vi "Runmin1.vi"(9 "循环次数 i":i32, 10 "Queue1":T2, 11 "prodatascan":T1) -> (1 "runMin":dbl, 2 "AD":dbl)   [LabVIEW 2018]
uses:
  Initialize/CreateQueue/AllDataQueue.ctl
  Initialize/CreateQueue/SocketQueue.ctl
  Initialize/CreateQueue/LogDataQueue.ctl
  Initialize/CreateQueue/ProDataQueue.ctl
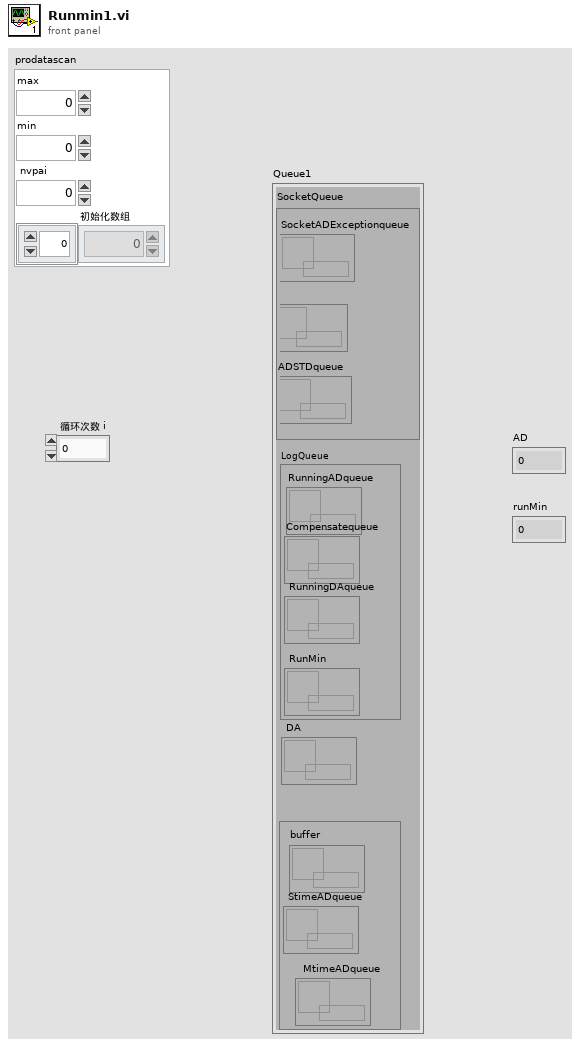
[diagram p1: front panel]
types:
  T1 = cluster{"max":dbl, "min":dbl, " nvpai":dbl, "初始化数组":dbl[]}
  T2 = typedef "AllDataQueue.ctl" = cluster{"SocketQueue":T3, "LogQueue":T4, " DA":refnum<queue>, "ProQueue":T5}
  T3 = typedef "SocketQueue.ctl" = cluster{"ADSTDqueue ":refnum<queue>, "SocketADExceptionqueue":refnum<queue>, "  SocketAD":refnum<queue>}
  T4 = typedef "LogDataQueue.ctl" = cluster{"RunningADqueue":refnum<queue>, "Compensatequeue":refnum<queue>, " RunningDAqueue":refnum<queue>, " RunMin":refnum<queue>}
  T5 = typedef "ProDataQueue.ctl" = cluster{"buffer ":refnum<queue>, " StimeADqueue":refnum<queue>, "  MtimeADqueue":refnum<queue>}
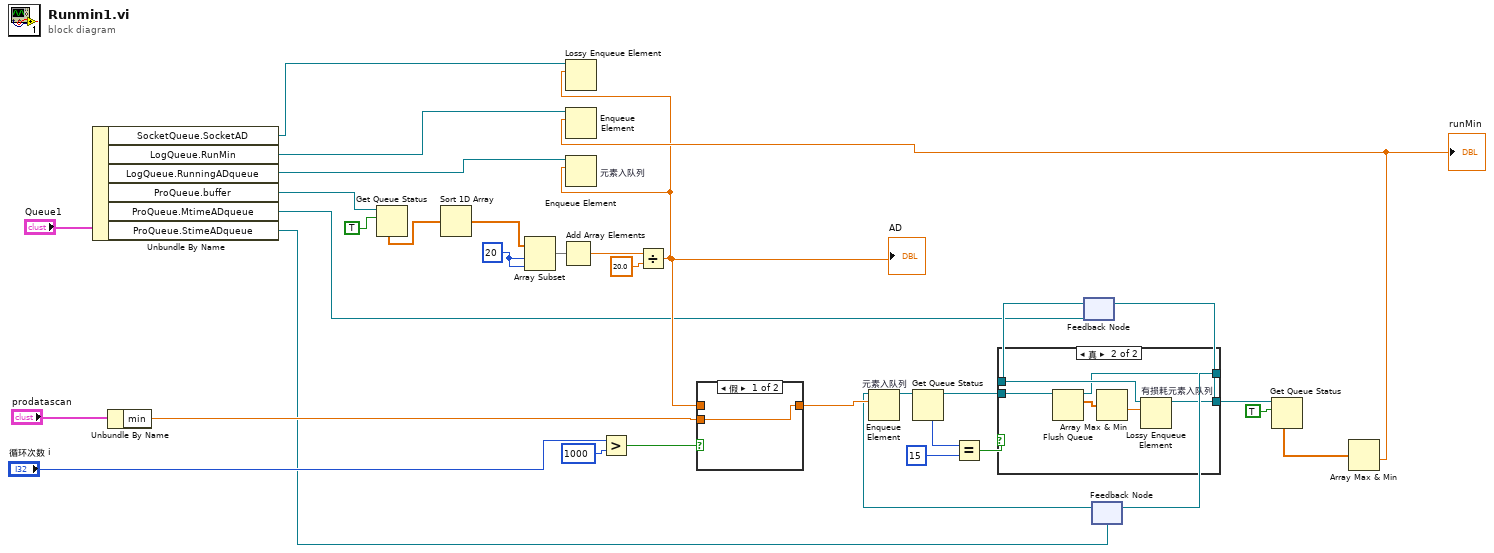
[diagram p0: block diagram]
diagram:
  w3 = 20 ("索引")
  n1 = Unbundle By Name("Queue1") -> ("SocketQueue.SocketAD"=w9:refnum<queue>, "LogQueue.RunMin"=w14:refnum<queue>, "LogQueue.RunningADqueue"=w13:refnum<queue>, "ProQueue.buffer"=w15:refnum<queue>, "ProQueue.MtimeADqueue"=w2:refnum<queue>, "ProQueue.StimeADqueue"=w1:refnum<queue>)
  n2 = Unbundle By Name("prodatascan") -> ("min"=w12:dbl)
  n3 = Get Queue Status(queue=w15, return elements? (F)=TRUE ("返回元素？(F)")) -> (elements=w4:dbl[])  [unwired: 1 in, 7 out]
  n4 = Sort 1D Array(array=w4) -> (sorted array=w10:dbl[])
  n5 = Array Subset(array=w10, index=w3, length=w3) -> (w30:dbl[])
  n6 = Add Array Elements(numeric array=w30) -> (sum=w31:dbl)
  n7 = Greater?(x="循环次数 i", y=1000) -> (0:w27:bool)
  n8 = Divide(x=w31, y=20.0) -> (x/y=w8:dbl)
  "AD" <- w8
  n9 = Lossy Enqueue Element(queue=w9, element=w8) -> ()  [unwired: 1 in, 4 out]
  n10 = Enqueue Element "元素入队列"(queue=w13, element=w8) -> ()  [unwired: 2 in, 3 out]
  n11 = case shown="假" w27 {
    tunnel: [w34 w35] -> w28
    tunnel: w8 -> [_ w35]
    tunnel: w12 -> [w34 _]
    frame False {
    }
    frame True {
    }
  }
  n12 = feedback #1(w2) -> (w23:refnum<queue>)
  n13 = feedback #2(w1) -> (w21:refnum<queue>)
  n14 = Enqueue Element "元素入队列"(queue=w21, element=w28) -> (queue out=w17:refnum<queue>)  [unwired: 2 in, 2 out]
  n15 = Get Queue Status(queue=w17) -> (queue out=w20:refnum<queue>, # elements in queue=w18:i32)  [unwired: 2 in, 6 out]
  n16 = Equal?(x=w18, y=15) -> (x = y?=w19:bool)
  n17 = case shown="真" w19 {
    tunnel: w20 -> [w37 w43]
    tunnel: w23 -> [w36 w40]
    tunnel: [w37 w39] -> w22
    tunnel: [w36 w38] -> w25
    frame False {
    }
    frame True {
      n18 = Flush Queue(queue=w43) -> (queue out=w39:refnum<queue>, remaining elements=w42:dbl[])  [unwired: 1 in, 1 out]
      n19 = Array Max & Min(array=w42) -> (min value=w41:dbl)  [unwired: 3 out]
      n20 = Lossy Enqueue Element "有损耗元素入队列"(queue=w40, element=w41) -> (queue out=w38:refnum<queue>)  [unwired: 1 in, 3 out]
    }
  }
  n21 = feedback-in #1(w25) -> ()
  n22 = feedback-in #2(w22) -> ()
  n23 = Get Queue Status(queue=w25, return elements? (F)=TRUE ("返回元素？(F)")) -> (elements=w26:dbl[])  [unwired: 1 in, 7 out]
  n24 = Array Max & Min(array=w26) -> (min value=w11:dbl)  [unwired: 3 out]
  "runMin" <- w11
  n25 = Enqueue Element(queue=w14, element=w11) -> ()  [unwired: 2 in, 3 out]
